vi "Execution Mode Type String.vi"(11 "CD Template":refnum<class "NIVS_CD Template.lvclass">) -> (2 "Execution Mode Type String":string)   [LabVIEW 2015, in "NIVS_CD Template.lvclass"]
uses:
  NIVS_CD Template.lvclass
  NIVS_Consolidated_CDW_MetaDataObj/Common.ctl
  NIVS_Consolidated_CDW_MetaDataObj/NIVS_Consolidated_CDW_MetaDataObj.lvclass
  NIVS_Consolidated_CDW_MetaDataObj/Common.vi
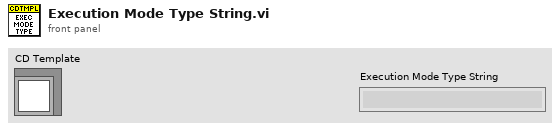
[diagram p1: front panel]
types:
  T1 = typedef "NIVS_Consolidated_CDW_MetaDataObj.lvclass/Common.ctl" = enum16{"ProjectName", "TemplatesFolderName", "ProjectTemplatePathAndName", "TimingAndSyncFolderName", "CustomDeviceFolderName", "PathToTemplates"}
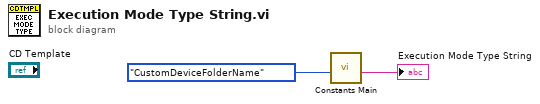
[diagram p0: block diagram]
diagram:
  n1 = call-poly "Constants Main.vi"("Action"=Common."CustomDeviceFolderName") -> ("Output"=→"Execution Mode Type String":string)  [unwired: 10 in]
